vi "ILAB_RemoteAppRef.vi"(2 "port":u32, 3 "machineName":string) -> (0 "errorOut":errorcluster, 1 "appReference":refnum<vi>)   [LabVIEW 2009]
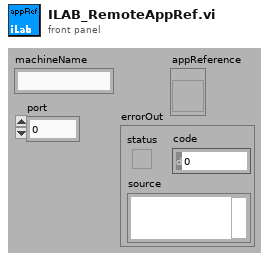
[diagram p1: front panel]
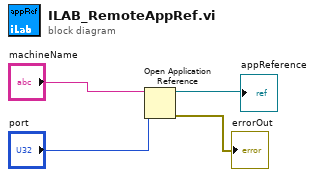
[diagram p0: block diagram]
diagram:
  n1 = Open Application Reference(10:"port", 11:"machineName") -> (0:→"errorOut":errorcluster, 3:→"appReference":refnum<vi>)  [unwired: 1 in, 1 out]
